vi "Write Display Settings 2 File.vi"(8 "error in":errorcluster, 10 "Saved ROIs":T3[](array[typedef]), 11 "State":T4 {"ROI"."Contours"."Type" items=["No Selection", "Point", "Line", "Rectangle", "Oval", "Polygon", "Freehand Region", "Annulus", "Unused2", "Unused3", "Broken Line", "Freehand Line", "Rotated Rectangle"]}) -> (0 "error out":errorcluster)   [LabVIEW 2009, in "POLARIS IMAQ Display.xctl"]
uses:
  POLARIS IMAQ Display.xctl
  State.ctl
  IMAQdx Cam/IMAQdx Cam.lvclass
  Properties/ImageSource.ctl
  <vilib>/vision/Image Controls.llb/IMAQ Image.ctl
  DisplaySettings.ctl
  Named ROI.ctl
panel:
  in  "Display settings":T1={"Min. Thresh."=0.0, "X"=0.0, "Y"=0.0, "ShowLineout"=FALSE, "ScaleParts"=10, "ShowLegende"=FALSE, "Target Cross"=FALSE, "Centroid Cross"=FALSE, "Target color"=16777226, "Centroid color"=16711680}
  in  "ROI":T2 {"Contours"."Type" items=["No Selection", "Point", "Line", "Rectangle", "Oval", "Polygon", "Freehand Region", "Annulus", "Unused2", "Unused3", "Broken Line", "Freehand Line", "Rotated Rectangle"]}
  in  "Calibration mm/px":dbl
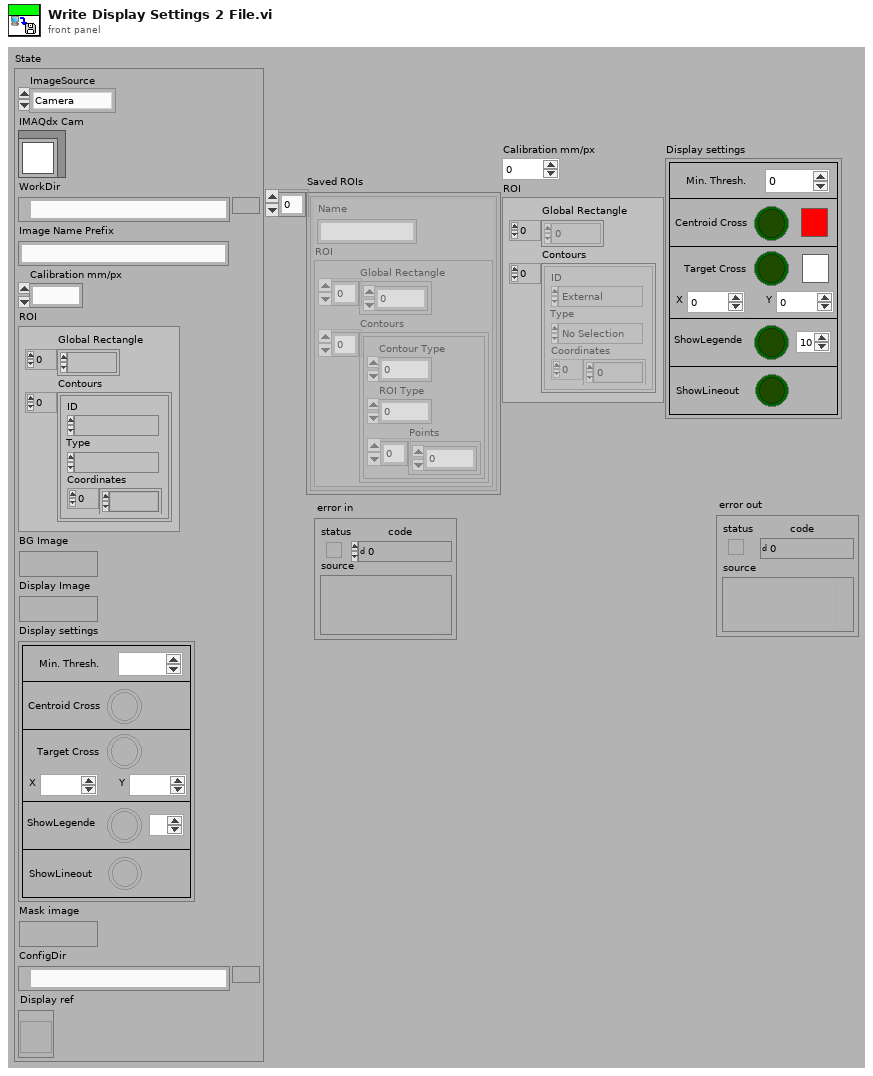
[diagram p1: front panel]
types:
  T1 = typedef "POLARIS IMAQ Display.xctl/DisplaySettings.ctl" = cluster{"Min. Thresh.":sgl, "X":dbl, "Y":dbl, "ShowLineout":bool, "ScaleParts":i32, "ShowLegende":bool, "Target Cross":bool, "Centroid Cross":bool, "Target color":u32, "Centroid color":u32}
  T2 = typedef "ROI Descriptor" = cluster{"Global Rectangle":i32[], "Contours":cluster{"ID":enum32{"External", "Internal"}, "Type":u32, "Coordinates":i32[]}[]}
  T3 = typedef "POLARIS IMAQ Display.xctl/Named ROI.ctl" = cluster{"ROI":cluster{"Global Rectangle":i32[], "Contours":cluster{"Contour Type":u32, "ROI Type":u32, "Points":i32[]}[]}, "Name":string}
  T4 = typedef "POLARIS IMAQ Display.xctl/State.ctl" = cluster{"ImageSource":T5, "IMAQdx Cam":refnum<class "IMAQdx Cam.lvclass">, "WorkDir":path, "Image Name Prefix":string, "Calibration mm/px":dbl, "ROI":T2, "BG Image":T6, "Display Image":T6, "Display settings":T1, "Mask image":T6, "ConfigDir":path, "Display ref":refnum<vi>}
  T5 = typedef "POLARIS IMAQ Display.xctl/ImageSource.ctl" = enum16{"Camera", "File"}
  T6 = typedef "IMAQ Image.ctl" = refnum<image>
  T7 = typedef "IMAQdx.ctl" = refnum<k21>
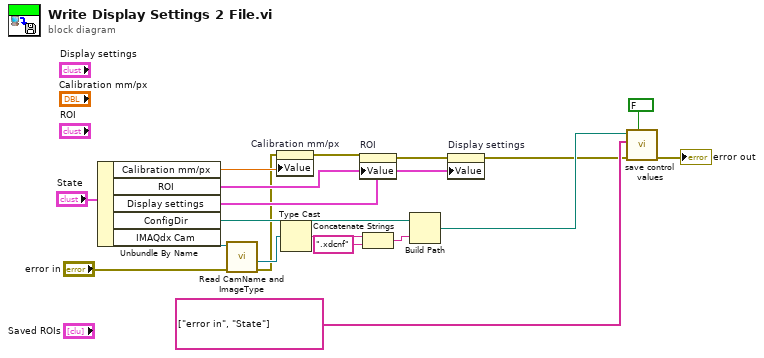
[diagram p0: block diagram]
diagram:
  n1 = Unbundle By Name("State") -> ("Calibration mm/px"=w7:dbl, "ROI"=w6:T2, "Display settings"=w5:T1, "ConfigDir"=w14:path, "IMAQdx Cam"=w17:refnum<class "IMAQdx Cam.lvclass">)
  n2 = call-dynamic "Read CamName and ImageType.vi"("error in (no error)"="error in", "IMAQdx Cam in"=w17) -> ("error out"=w2:errorcluster, "Camera"=w13:T7)  [unwired: 6 in, 2 out]
  n3 = property on="Calibration mm/px" class="DigNum (strict)"(error in=w2, "Value"=w7) -> (error out=w4:errorcluster)  [unwired: 1 in, 1 out]
  n4 = Type Cast(x=w13) -> (*(type *) &x=w12:string)  [unwired: 1 in]
  n5 = property on="ROI" class="Clust (strict)"(error in=w4, "Value"=w6) -> (error out=w3:errorcluster)  [unwired: 1 in, 1 out]
  n6 = Concatenate Strings(w12, ".xdcnf" ("string")) -> (w9:string)
  n7 = Build Path(base path=w14, name or relative path=w9) -> (appended path=w15:path)
  n8 = property on="Display settings" class="Clust (strict)"(error in=w3, "Value"=w5) -> (error out=w1:errorcluster)  [unwired: 1 in, 1 out]
  n9 = call "save control values.vi"("Append timestamp (true)"=FALSE, "error in"=w1, "Dont save"=string[] ["error in", "State"], "Path"=w15) -> ("error out"=→"error out":errorcluster)  [unwired: 4 in, 1 out]
